vi "F020_time32_get.vi"(8 "error in":errorcluster, 10 "Cluster":cluster{"ADDRESS":u8}={"ADDRESS"=170}, 11 "COM in":string="COM4") -> (0 "error out":errorcluster={"status"=TRUE, "code"=-1073807343, "source"=""}, 2 "RUNTIME out":u32, 3 "COM out":string="COM4")   [LabVIEW 2016]
doc: "This example performs a serial port write and a serial port read. The parameters set for the serial port must match the parameters of the connected instrument or device. The VISA Configure Serial Port VI sets the configuration parameters. The front panel displays the controls used to configure the basic parameters, such as baud rate, data bits, and parity. The VI passes the VISA resource name to other VIs that perform operations on that VISA resource. The VISA Write function sends a command to the serial device and the VISA Read function returns data based on the command. The VISA Close function then closes the reference to the serial device. It is important to close the reference; otherwise, further communication through that port might not be possible."
panel:
  # "loopback: <xxAABB>\nwr_dout:   <xxAA11aabbccdd> aa=ch, bb=val, ccdd=timeout[sec]\nrd_ain:      <xxAA13aa> -> {qqww}"
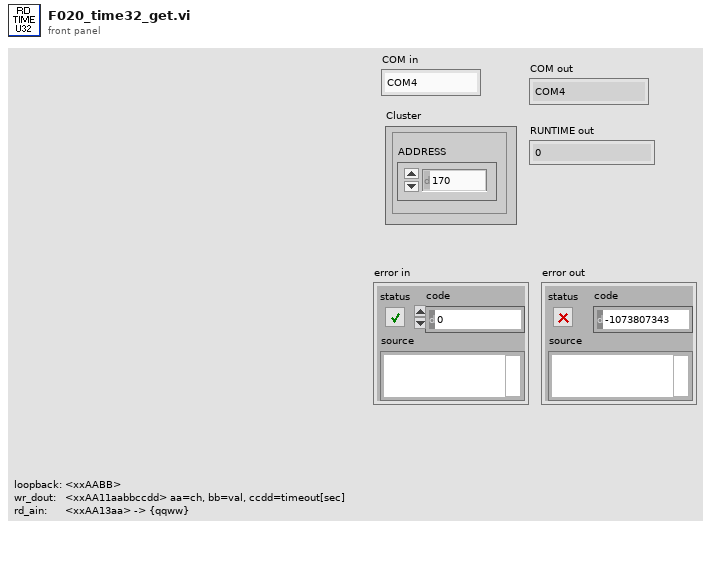
[diagram p1: front panel]
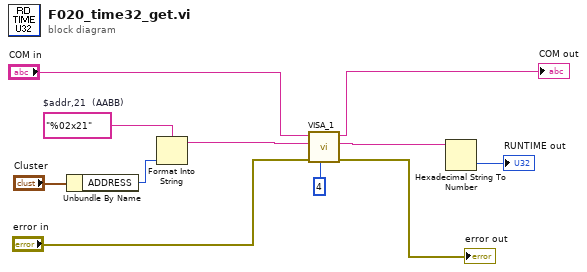
[diagram p0: block diagram]
diagram:
  w7 = "%02x21"  # $addr,21  (AABB)
  n1 = Unbundle By Name("Cluster") -> ("ADDRESS"=w4:u8)
  n2 = Format Into String(format string=w7, w4) -> (resulting string=w3:string)  [unwired: 2 in, 1 out]
  n3 = call "VISA_1.vi"("delay[ms]"=u32 4, "error in"="error in", "wr_buf"=w3, "COM in"="COM in") -> ("error out"=→"error out":errorcluster, "rx_buf"=w5:string, "COM out"=→"COM out":string)  [unwired: 4 in, 1 out]
  n4 = Hexadecimal String To Number(string=w5) -> (number=→"RUNTIME out":u32)  [unwired: 2 in, 1 out]
